vi "Convert BC Section From Parameter List.vi"(0 "BC Section String":string) -> (4 "BC Messages":T1[](array[typedef]))   [LabVIEW 2011, in "AIT 1553 Custom Device.lvlib"]
uses:
  AIT 1553 Custom Device.lvlib
  Controls/1553_BC_Message.ctl
  Controls/1553 Param.ctl
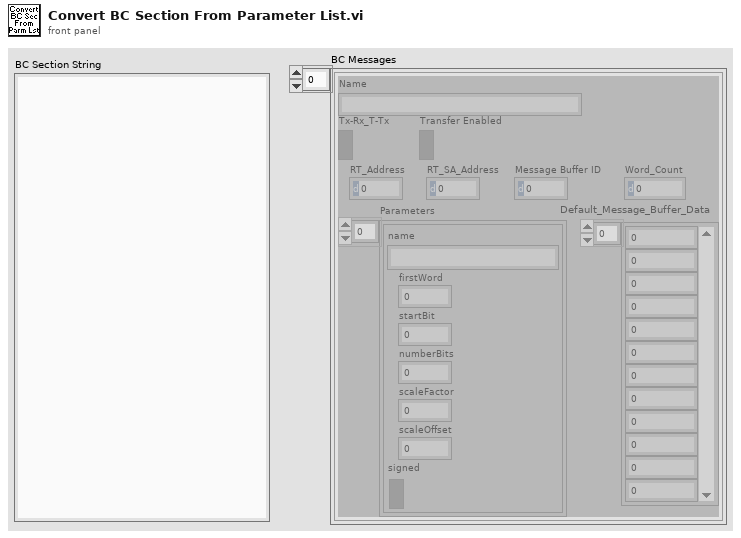
[diagram p1: front panel]
types:
  T1 = typedef "AIT 1553 Custom Device.lvlib/1553_BC_Message.ctl" = cluster{"Name":string, "Tx-Rx_T-Tx":bool, "RT_Address":u8, "RT_SA_Address":u8, "Parameters":T2[], "Transfer Enabled":bool, "Message Buffer ID":u16, "Default_Message_Buffer_Data":u16[], "Word_Count":u8}
  T2 = typedef "AIT 1553 Custom Device.lvlib/1553 Param.ctl" = cluster{"name":string, "firstWord":i32, "startBit":i32, "numberBits":i32, "scaleFactor":dbl, "scaleOffset":dbl, "signed":bool}
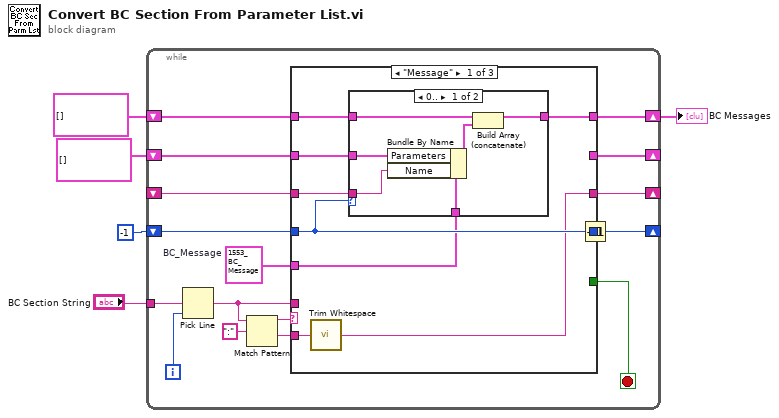
[diagram p0: block diagram]
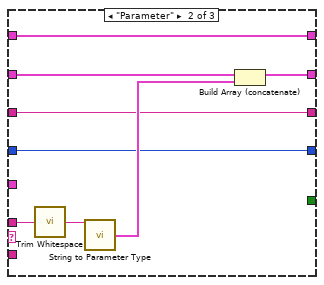
[diagram p3: hidden frame]
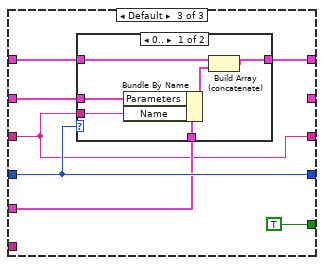
[diagram p4: hidden frame]
diagram:
  n1 = while {
    tunnel: "BC Section String" -> [w21]
    shift-right: [w17] -> w2
    shift-left: T1[] [] -> [w18]
    shift-right: [w15] -> _
    shift-left: -1 -> [w16]
    shift-right: [w12] -> _
    shift-left: T2[] [] ("Parameters") -> [w13]
    shift-right: [w10] -> _
    shift-left: _ -> [w9]
    i -> [w7]
    stop <- w8 stop-if-true
    w19 = T1 {"Name"="Gun_One", "Tx-Rx_T-Tx"=FALSE, "RT_Address"=11, "RT_SA_Address"=10, "Parameters"=[{"name"="Data_01", "firstWord"=8, "startBit"=0, "numberBits"=8, "scaleFactor"=1.0, "scaleOffset"=0.0, "signed"=FALSE}], "Transfer Enabled"=TRUE, "Message Buffer ID"=0, "Default_Message_Buffer_Data"=[0, 1, 2, 3, 4, 5, 6, 7, 8, 9, 10, 11, 12, 13, 14, 15, 16, 17, 18, 19, 20, 21, 22, 23, 24, 25, 26, 27, 28, 29], "Word_Count"=30}  # BC_Message
    n2 = Pick Line(multi-line string=w21, line index=w7) -> (output string=w14:string)  [unwired: 1 in]
    n3 = Match Pattern(string=w14, regular expression=":") -> (before substring=w6:string, after substring=w11:string)  [unwired: 1 in, 2 out]
    n4 = case shown="\"Message\"" w6 {
      tunnel: w19 -> [w23 _ w49]
      tunnel: w18 -> [w27 w44 w52]
      tunnel: [w25 w44 w48] -> w17
      tunnel: w16 -> [w28 w40 w50]
      tunnel: [w30 w40 w50] -> w15
      tunnel: w14 -> [_ w45 _]
      tunnel: w13 -> [w22 w43 w51]
      tunnel: [_ w42 _] -> w12
      tunnel: w11 -> [w29 _ _]
      tunnel: [w26 w38 w46] -> w10
      tunnel: w9 -> [w24 w38 w46]
      tunnel: [_ _ TRUE] -> w8
      frame "Message" {
        n5 = call <vilib>:"Trim Whitespace.vi"("string"=w29) -> ("trimmed string"=w26:string)  [unwired: 1 in]
        n6 = case shown="0.." w28 {
          tunnel: [w31 w37] -> w25
          tunnel: w27 -> [w34 w37]
          tunnel: w24 -> [w36 _]
          tunnel: w23 -> [w35 _]
          tunnel: w22 -> [w32 _]
          frame 0.. {
            n7 = Bundle By Name(cluster=w35, "Parameters"=w32, "Name"=w36) -> (w33:T1)
            n8 = Build Array (concatenate)(w34, w33) -> (w31:T1[])
          }
          frame Default {
          }
        }
        n9 = Increment(x=w28) -> (x+1=w30:i32)
      }
      frame "Parameter" {
        n10 = call <vilib>:"Trim Whitespace.vi"("string"=w45) -> ("trimmed string"=w39:string)  [unwired: 1 in]
        n11 = call "String to Parameter Type.vi"("String in"=w39) -> ("Parameter-1553"=w41:T2)  [unwired: 12 in, 2 out]
        n12 = Build Array (concatenate)(w43, w41) -> (w42:T2[])
      }
      frame Default {
        n13 = case shown="0.." w50 {
          tunnel: [w53 w59] -> w48
          tunnel: w52 -> [w56 w59]
          tunnel: w46 -> [w58 _]
          tunnel: w49 -> [w57 _]
          tunnel: w51 -> [w54 _]
          frame 0.. {
            n14 = Bundle By Name(cluster=w57, "Parameters"=w54, "Name"=w58) -> (w55:T1)
            n15 = Build Array (concatenate)(w56, w55) -> (w53:T1[])
          }
          frame Default {
          }
        }
      }
    }
  }
  "BC Messages" <- w2
